vi "Spawn Win Msg Daemon.vi"(4 "error in (no error)":errorcluster, 5 "Messages (none)":u32[](array[numeric]), 6 "WinMsg Event":refnum<user-event>, 7 "VI Refnum":refnum<vi>) -> (0 "error out":errorcluster, 3 "dup VI Refnum":refnum<vi>)   [LabVIEW 2011]
uses:
  Win Msg.ctl
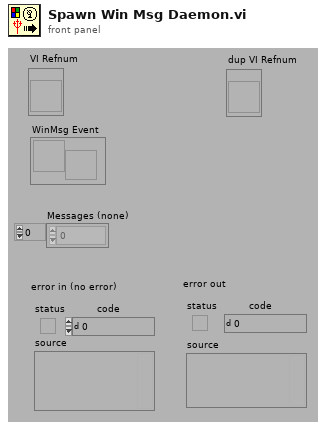
[diagram p1: front panel]
types:
  T1 = typedef "Rendezvous RefNum" = refnum<k1>
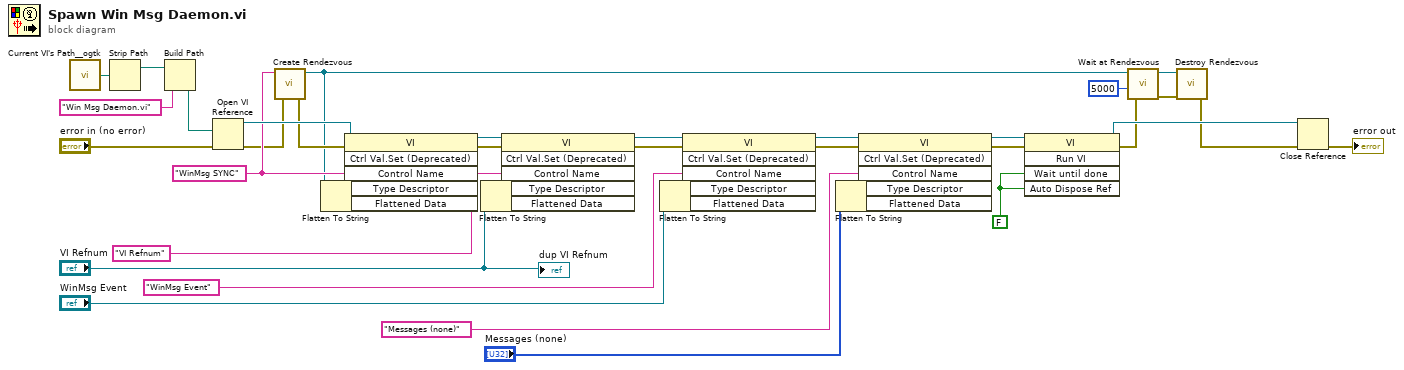
[diagram p0: block diagram]
diagram:
  w20 = FALSE
  w33 = "WinMsg SYNC" ("name or relative path")
  n1 = call <userlib>:"Current VI's Path__ogtk.vi"() -> ("Current VI's Path (+ Relative)"=w38:path)  [unwired: 1 out]
  n2 = Strip Path(path=w38) -> (stripped path=w37:path)  [unwired: 1 out]
  n3 = Build Path(base path=w37, name or relative path="Win Msg Daemon.vi") -> (appended path=w35:path)
  n4 = Open VI Reference(vi path=w35, error in (no error)="error in (no error)") -> (vi reference=w34:refnum<vi>, error out=w32:errorcluster)  [unwired: 4 out]
  n5 = call <vilib>:"Create Rendezvous.vi"("error in (no error)"=w32, "name (unnamed)"=w33) -> ("error out"=w31:errorcluster, "rendezvous"=w15:T1)  [unwired: 1 in, 3 out]
  n6 = Flatten To String(anything=w15) -> (data string=w29:string, type string=w30:i16[])  [unwired: 1 in, 3 out]
  n7 = invoke class="VI" method="Ctrl Val.Set (Deprecated)"(reference=w34, error in=w31, "Control Name"=w33, "Type Descriptor"=w30, "Flattened Data"=w29) -> (reference out=w27:refnum<vi>, error out=w28:errorcluster)  [unwired: 1 in, 4 out]
  n8 = Flatten To String(anything="VI Refnum") -> (data string=w25:string, type string=w26:i16[])  [unwired: 1 in, 3 out]
  n9 = invoke class="VI" method="Ctrl Val.Set (Deprecated)"(reference=w27, error in=w28, "Control Name"="VI Refnum" ("name or relative path"), "Type Descriptor"=w26, "Flattened Data"=w25) -> (reference out=w23:refnum<vi>, error out=w24:errorcluster)  [unwired: 1 in, 4 out]
  n10 = Flatten To String(anything="WinMsg Event") -> (data string=w21:string, type string=w22:i16[])  [unwired: 1 in, 3 out]
  n11 = invoke class="VI" method="Ctrl Val.Set (Deprecated)"(reference=w23, error in=w24, "Control Name"="WinMsg Event" ("name or relative path"), "Type Descriptor"=w22, "Flattened Data"=w21) -> (reference out=w5:refnum<vi>, error out=w6:errorcluster)  [unwired: 1 in, 4 out]
  n12 = Flatten To String(anything="Messages (none)") -> (data string=w8:string, type string=w7:i16[])  [unwired: 1 in, 3 out]
  n13 = invoke class="VI" method="Ctrl Val.Set (Deprecated)"(reference=w5, error in=w6, "Control Name"="Messages (none)" ("name or relative path"), "Type Descriptor"=w7, "Flattened Data"=w8) -> (reference out=w3:refnum<vi>, error out=w4:errorcluster)  [unwired: 1 in, 4 out]
  n14 = invoke class="VI" method="Run VI"(reference=w3, error in=w4, "Wait until done"=w20, "Auto Dispose Ref"=w20) -> (reference out=w19:refnum<vi>, error out=w14:errorcluster)  [unwired: 1 in, 3 out]
  n15 = call <vilib>:"Wait at Rendezvous.vi"("error in (no error)"=w14, "ms timeout (-1)"=5000, "rendezvous"=w15) -> ("error out"=w18:errorcluster, "rendezvous out"=w17:T1)  [unwired: 3 out]
  n16 = call <vilib>:"Destroy Rendezvous.vi"("error in (no error)"=w18, "rendezvous"=w17) -> ("error out"=w10:errorcluster)  [unwired: 5 out]
  n17 = Close Reference(reference=w19, error in (no error)=w10) -> (error out=→"error out":errorcluster)
  "dup VI Refnum" <- "VI Refnum"
